vi "init_actuator.vi"(8 "error in":errorcluster, 11 "Actuator cluster in":T1={"Actuator COM"="COM14", "Actuator type"=enum."Scientifica"}) -> (0 "error out":errorcluster, 2 "initialization error":bool, 3 "Actuator cluster out":T1={"Actuator COM"="COM14", "Actuator type"=enum."Scientifica"})   [LabVIEW 2015]
uses:
  controls/actuator_type.ctl
  controls/actuator_cluster.ctl
panel:
  # "INIT ACTUATOR"
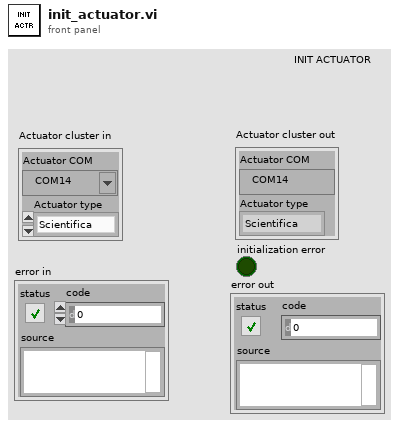
[diagram p1: front panel]
types:
  T1 = typedef "actuator_cluster.ctl" = cluster{"Actuator COM":refnum<visa-resource-name>, "Actuator type":T2}
  T2 = typedef "actuator_type.ctl" = enum16{"Scientifica", "Sutter", "Demo", "Off"}
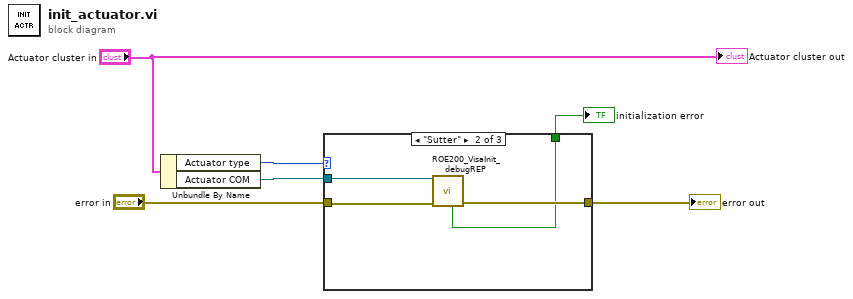
[diagram p0: block diagram]
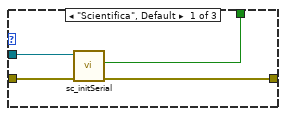
[diagram p2: hidden frame]
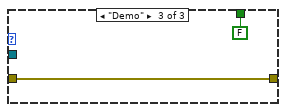
[diagram p3: hidden frame]
diagram:
  n1 = Unbundle By Name("Actuator cluster in") -> ("Actuator type"=w6:T2, "Actuator COM"=w4:refnum<visa-resource-name>)
  n2 = case shown="\"Sutter\"" w6 {
    tunnel: "error in" -> [w9 w13 w15]
    tunnel: w4 -> [w10 w14 _]
    tunnel: [w8 w12 w15] -> w1
    tunnel: [w7 w11 FALSE ("error in initialization")] -> w3
    frame "Scientifica", Default {
      n3 = call "sc_initSerial.vi"("error in (no error)"=w9, "VISA resource name"=w10) -> ("error out"=w8:errorcluster, "initialization error"=w7:bool)  [unwired: 7 in, 1 out]
    }
    frame "Sutter" {
      n4 = call "ROE200_VisaInit_debugREP.vi"("error in (no error)"=w13, "VISA resource name"=w14) -> ("error out"=w12:errorcluster, "error in initialization"=w11:bool)  [unwired: 7 in, 1 out]
    }
    frame "Demo" {
    }
  }
  "initialization error" <- w3
  "error out" <- w1
  "Actuator cluster out" <- "Actuator cluster in"
